vi "Pockels-Bundle funct acq simulation inputs.vi"(9 "AOL_Globals":T2={"Imaging Protocol"=enum."AOL Z-Stack", "Number of POI"=0, "Number of Miniscans"=0, "Number of Trials"=0, "Number of Cycles "=0, "# Averaged Frames"=0, "Laser power (%)"=0, "Pockels"=0.0, "Acquisition Length (sec)"=0.0, "Fill time (us)"=0.0, "POI Dwell time (us)"=0.0, "Miniscan Dwell time per pixel (us)"=0.0, "PMT 1"=0.0, "PMT 2"=0.0, "Back Apperture"=0.0, "Frame Size"=0, "Center Frequency"=0.0, "Field of View"=0.0, "DwellTime (us)"=0.0, "Wavelength (nm)"=0.0, "Zoom"=0.0, "AOL Z"=0.0, "AOL Mode"=enum."Raster", "GridXY"=0.0, "GridZ"=0.0, "TriggerPeriod (sec)"=0.0, "Number of Pixels in Miniscan"=0, "Experiment folder path"=path "", "X centre"=0.0, "Y centre"=0.0, "Angle (degrees)"=0.0, "Plane Mode"=0, "Threshold"=[], "Regenerate Chirps"=FALSE, "Rectangle ROI length (pixels)"=0, "Rectangle ROI height (pixels)"=0, "AOD fill"=0, "Samples Wait after Trigger"=0, "StartUp Delay"=0, "Slip Cycle"=163840, "Add Cycle"=FALSE} {"Plane Mode" items=["XY Plane"]; "Frame Size" items=["100X100"=100, "128X128"=128, "200X200"=200, "256X256"=256, "512X512"=512, "1024x1024"=1024, "2048x2048"=2048]; "Back Apperture" format="%#.6g"; "Pockels" format="%#.6g"; "PMT 2" format="%#.6g"; "PMT 1" format="%#.6g"; "Angle (degrees)" format="%#.6g"; "POI Dwell time (us)" format="%#.6g"}, 11 "Simulation inputs cluster":T7={"Dwell time (us) -Manual"=4.2, "Simulated number of POI"=8, "Bypass"=FALSE, "Pockels \"Low\" time (us)"=20.0, "AO Sample Clock Rate (samples/sec)"=0.0, "Control system simulated waveform"=FALSE} {"AO Sample Clock Rate (samples/sec)" format="%#_6f"; "Dwell time (us) -Manual" min=0.05 max=10.0 step=0.1 format="%#.1fus"}) -> (1 "Array":T1[](array[typedef]) {"ROI group ID" format="%#_6f"; "Laser Power (%)" format="%#_6f"; "Zoom" format="%#_6f"; "Frame Size" format="%#_6f"; "Number of lines" format="%#_6f"; "Composite ID" format="%#_6f"; "Angle (deg)" format="%#_6f"; "ROI Time (ns)" format="%#_6f"; "ROI ID" format="%#_6f"; "Pixels in ROI" format="%#_6f"; "ROI index" format="%#_6f"; "Z stop" format="%#_6f"; "Y stop" format="%#_6f"; "X stop" format="%#_6f"; "Z start" format="%#_6f"; "X start" format="%#_6f"; "Y start" format="%#_6f"}, 3 "Simulated number of POI":i32)   [LabVIEW 2013]
uses:
  Typedefs/Pockels-Funct acq simulation inputs cluster.ctl
  Typedefs/Controls/AOL_Globals.ctl
  Typedefs/Imaging Protocols enum.ctl
  Typedefs/Frame Size.ctl
  Typedefs/AOL modes.ctl
  Typedefs/Plane Mode.ctl
  User Interface/Visualisation/Functional Imaging Viewer/Typedefs/ROI parameters data type.ctl
  Global Variables/General Globals.vi
  Globals/gl_Pockels control globals.vi
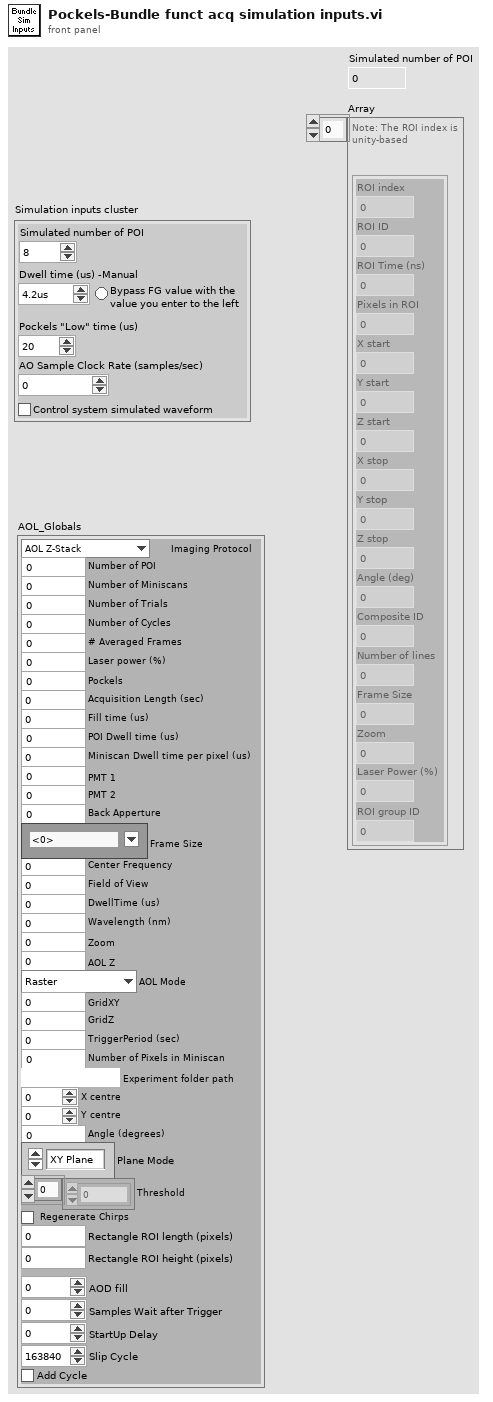
[diagram p1: front panel]
types:
  T1 = typedef "ROI parameters data type.ctl" = cluster{"ROI index":dbl, "ROI ID":dbl, "ROI Time (ns)":dbl, "Pixels in ROI":dbl, "X start":dbl, "Y start":dbl, "Z start":dbl, "X stop":dbl, "Y stop":dbl, "Z stop":dbl, "Angle (deg)":dbl, "Composite ID":dbl, "Number of lines":dbl, "Frame Size":dbl, "Zoom":dbl, "Laser Power (%)":dbl, "ROI group ID":dbl}
  T2 = typedef "AOL_Globals.ctl" = cluster{"Imaging Protocol":T3, "Number of POI":u16, "Number of Miniscans":u16, "Number of Trials":u16, "Number of Cycles ":u64, "# Averaged Frames":u16, "Laser power (%)":u8, "Pockels":dbl, "Acquisition Length (sec)":dbl, "Fill time (us)":dbl, "POI Dwell time (us)":dbl, "Miniscan Dwell time per pixel (us)":dbl, "PMT 1":dbl, "PMT 2":dbl, "Back Apperture":dbl, "Frame Size":T4, "Center Frequency":dbl, "Field of View":dbl, "DwellTime (us)":dbl, "Wavelength (nm)":dbl, "Zoom":dbl, "AOL Z":dbl, "AOL Mode":T5, "GridXY":dbl, "GridZ":dbl, "TriggerPeriod (sec)":dbl, "Number of Pixels in Miniscan":u16, "Experiment folder path":path, "X centre":dbl, "Y centre":dbl, "Angle (degrees)":dbl, "Plane Mode":T6, "Threshold":u16[], "Regenerate Chirps":bool, "Rectangle ROI length (pixels)":u16, "Rectangle ROI height (pixels)":u16, "AOD fill":u16, "Samples Wait after Trigger":u16, "StartUp Delay":i32, "Slip Cycle":u32, "Add Cycle":bool}
  T3 = typedef "Imaging Protocols enum.ctl" = enum16{"AOL Z-Stack", "Motor Z Stack", "Functional Acquisition", "Single Plane Acquisition", "Volume Acquisition", "Live Imaging", "Live Plane Imaging", "Live Volume Imaging"}
  T4 = typedef "Frame Size.ctl" = u16
  T5 = typedef "AOL modes.ctl" = enum16{"Raster", "Structural", "Pointing", "Mini Scan", "Alignment"}
  T6 = typedef "Plane Mode.ctl" = u16
  T7 = typedef "Pockels-Funct acq simulation inputs cluster.ctl" = cluster{"Dwell time (us) -Manual":dbl, "Simulated number of POI":i32, "Bypass":bool, "Pockels \"Low\" time (us)":dbl, "AO Sample Clock Rate (samples/sec)":dbl, "Control system simulated waveform":bool}
  T8 = cluster{"ZStack":cluster{"Zstart":dbl, "Zstop":dbl, "Zstep":dbl}, "Laser Power %":cluster{"@ Start":dbl, "@ Stop":dbl}}
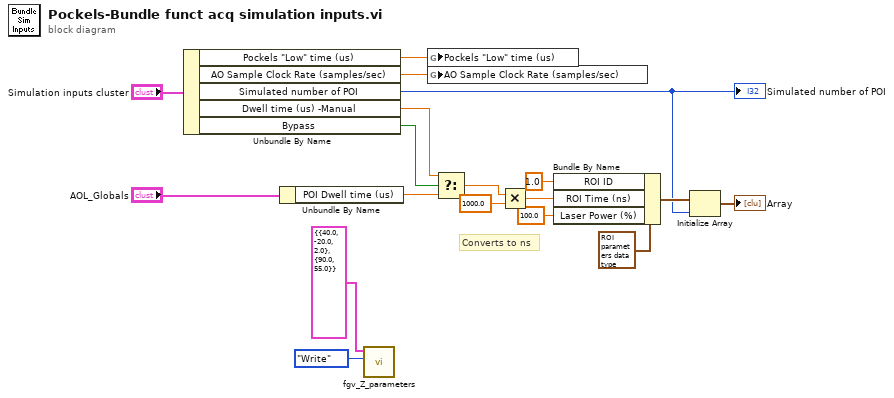
[diagram p0: block diagram]
diagram:
  # "Converts to ns"
  n1 = Unbundle By Name("Simulation inputs cluster") -> ("Pockels \"Low\" time (us)"=w16:dbl, "AO Sample Clock Rate (samples/sec)"=w17:dbl, "Simulated number of POI"=w4:i32, "Dwell time (us) -Manual"=w18:dbl, "Bypass"=w5:bool)
  "Simulated number of POI" <- w4
  n2 = Unbundle By Name("AOL_Globals") -> ("POI Dwell time (us)"=w15:dbl)
  n3 = call "fgv_Z_parameters.vi"("Function"=enum16{"Intialize", "Write", "Read", "Clear"}."Write", "Z Parameters"=T8 {"ZStack"={"Zstart"=40.0, "Zstop"=-20.0, "Zstep"=2.0}, "Laser Power %"={"@ Start"=90.0, "@ Stop"=55.0}}) -> ()  [unwired: 8 in, 2 out]
  n4 = global write "gl_Pockels control globals.vi" "Pockels \"Low\" time (us)"(w16) -> ()
  n5 = global write "General Globals.vi" "AO Sample Clock Rate (samples/sec)"(w17) -> ()
  n6 = Select(t=w18, s=w5, f=w15) -> (s? t:f=w13:dbl)
  n7 = Multiply(x=w13, y=1000.0) -> (x*y=w9:dbl)
  n8 = Bundle By Name(cluster=T1 {"ROI index"=0.0, "ROI ID"=0.0, "ROI Time (ns)"=0.0, "Pixels in ROI"=0.0, "X start"=0.0, "Y start"=0.0, "Z start"=0.0, "X stop"=0.0, "Y stop"=0.0, "Z stop"=0.0, "Angle (deg)"=0.0, "Composite ID"=0.0, "Number of lines"=0.0, "Frame Size"=0.0, "Zoom"=0.0, "Laser Power (%)"=0.0, "ROI group ID"=0.0} ("X-Y-Z coordinates"), "ROI ID"=1.0, "ROI Time (ns)"=w9, "Laser Power (%)"=100.0) -> (w11:T1)
  n9 = Initialize Array(w11, w4) -> (→"Array":T1[])
